vi "Mail Demo.vi"() -> ()   [LabVIEW 2012]
uses:
  MAIL.lvclass
panel:
  out "error out":errorcluster caption="错误输出"
  in  "Body":string
  in  "Subject":string
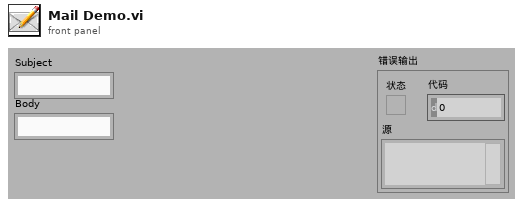
[diagram p1: front panel]
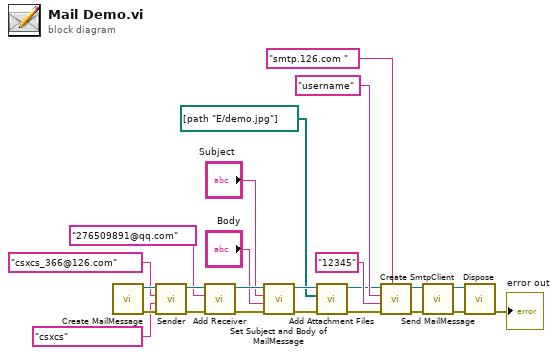
[diagram p0: block diagram]
diagram:
  n1 = call "Create MailMessage.vi"() -> ("error out"=w23:errorcluster, "Mail 输出"=w24:refnum<class "MAIL.lvclass">)  [unwired: 10 in]
  n2 = call "Sender.vi"("error in (no error)"=w23, "Sender Name"="csxcs", "Sender Address"="csxcs_366@126.com", "Mail 输入"=w24) -> ("error out"=w19:errorcluster, "Mail 输出"=w20:refnum<class "MAIL.lvclass">)  [unwired: 6 in]
  n3 = call "Add Receiver.vi"("error in (no error)"=w19, "Receiver Address"="276509891@qq.com", "Mail 输入"=w20) -> ("error out"=w13:errorcluster, "Mail 输出"=w14:refnum<class "MAIL.lvclass">)  [unwired: 7 in]
  n4 = call "Set Subject and Body of MailMessage.vi"("error in (no error)"=w13, "Body"="Body", "Subject"="Subject", "MAIL 输入"=w14) -> ("error out"=w4:errorcluster, "MAIL 输出"=w5:refnum<class "MAIL.lvclass">)  [unwired: 6 in]
  n5 = call "Add Attachment Files.vi"("error in (no error)"=w4, "Attachment Files"=path[] [path "E:/demo.jpg"], "MAIL 输入"=w5) -> ("error out"=w2:errorcluster, "MAIL 输出"=w3:refnum<class "MAIL.lvclass">)  [unwired: 7 in]
  n6 = call "Create SmtpClient.vi"("host"="smtp.126.com ", "error in (no error)"=w2, "password"="12345", "userName"="username", "MAIL 输入"=w3) -> ("error out"=w8:errorcluster, "MAIL 输出"=w9:refnum<class "MAIL.lvclass">)  [unwired: 5 in]
  n7 = call "Send MailMessage.vi"("error in (no error)"=w8, "MAIL 输入"=w9) -> ("error out"=w6:errorcluster, "MAIL 输出"=w7:refnum<class "MAIL.lvclass">)  [unwired: 8 in]
  n8 = call "Dispose.vi"("error in (no error)"=w6, "Mail 输入"=w7) -> ("error out"=→"error out":errorcluster)  [unwired: 8 in, 1 out]
